vi "SendQueryMsg.vi"(0 "VISAリソース名":refnum<visa-resource-name>, 5 "入力文字列":string, 7 "タイムアウト":u32, 9 "ターミネータ":string(combo)="\n", 11 "エラー入力":errorcluster) -> (6 "受信文字列":string, 15 "エラー出力":errorcluster)   [LabVIEW 2012]
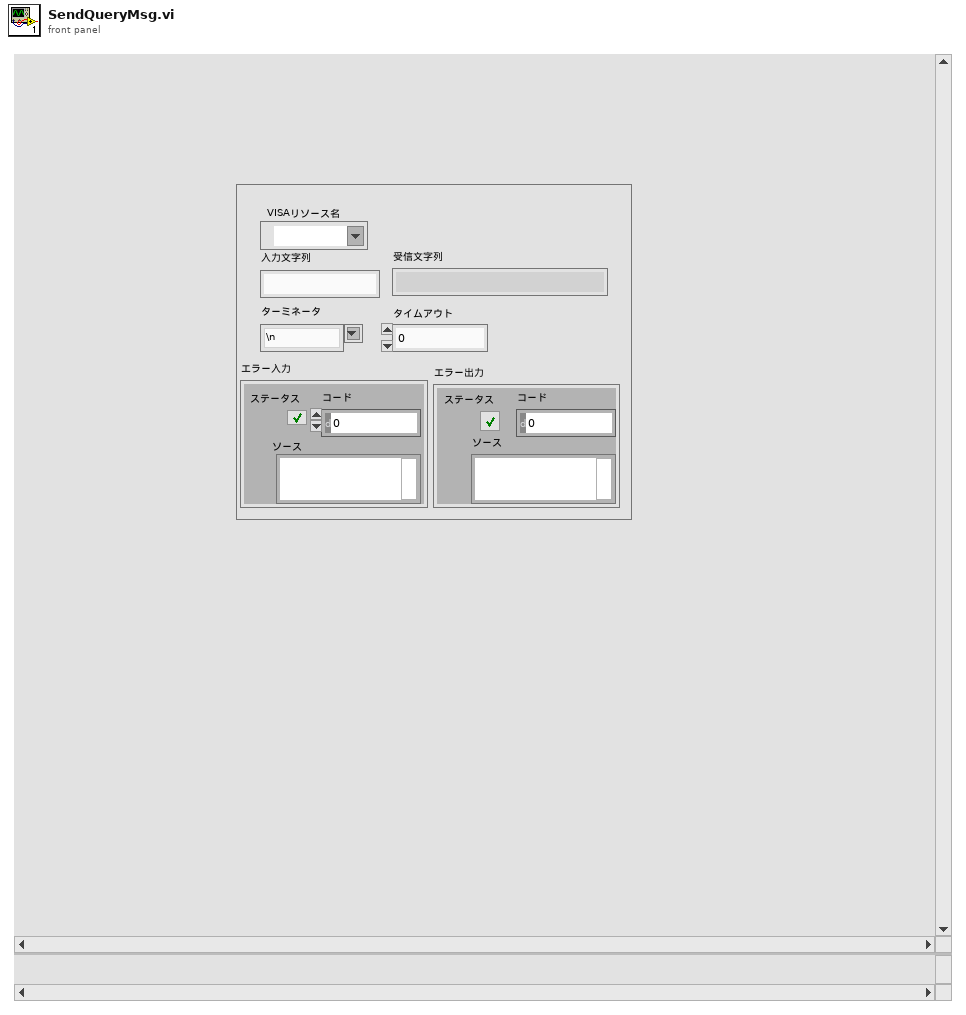
[diagram p1: front panel]
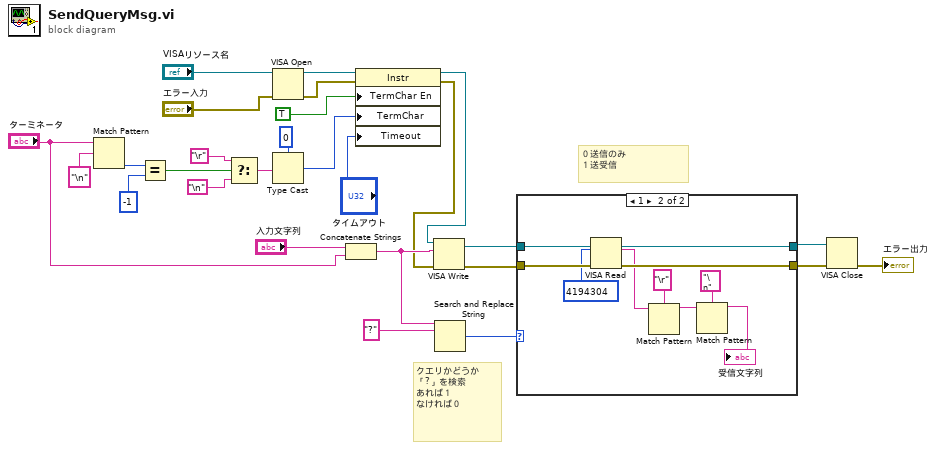
[diagram p0: block diagram]
diagram:
  # "０送信のみ\n１送受信"
  # "クエリかどうか\n「?」を検索\nあれば１\nなければ０"
  n1 = Match Pattern(string="ターミネータ", regular expression="\n" ("正規表現")) -> (offset past match=w3:i32)  [unwired: 1 in, 3 out]
  n2 = Equal?(x=w3, y=-1) -> (x = y?=w8:bool)
  n3 = Select(t="\r", s=w8, f="\n") -> (s? t:f=w9:string)
  n4 = VISA Open(error in (no error)="エラー入力", VISA resource name="VISAリソース名") -> (VISA resource name=w17:refnum<visa-resource-name>, error out=w14:errorcluster)  [unwired: 3 in]
  n5 = Type Cast(type=u8 0, x=w9) -> (*(type *) &x=w10:u8)
  n6 = Concatenate Strings("入力文字列", "ターミネータ") -> (w25:string)
  n7 = property class="Instr"(reference=w17, error in=w14, "TermChar En"=TRUE, "TermChar"=w10, "Timeout"="タイムアウト") -> (reference out=w16:refnum<visa-resource-name>, error out=w13:errorcluster)
  n8 = VISA Write(VISA resource name=w16, write buffer=w25, error in (no error)=w13) -> (VISA resource name out=w23:refnum<visa-resource-name>, error out=w21:errorcluster)  [unwired: 1 out]
  n9 = Search and Replace String(input string=w25, search string="?" ("検索文字列")) -> (number of replacements=w26:i32)  [unwired: 6 in, 3 out]
  n10 = case shown="1" w26 {
    tunnel: w21 -> [w28 w39]
    tunnel: [w29 w38] -> w24
    tunnel: w23 -> [w29 w37]
    tunnel: [w28 w35] -> w20
    frame 0, Default {
    }
    frame 1 {
      n11 = VISA Read(VISA resource name=w37, byte count=4194304, error in (no error)=w39) -> (VISA resource name out=w38:refnum<visa-resource-name>, read buffer=w31:string, error out=w35:errorcluster)  [unwired: 1 out]
      n12 = Match Pattern(string=w31, regular expression="\r") -> (before substring=w34:string)  [unwired: 1 in, 3 out]
      n13 = Match Pattern(string=w34, regular expression="\n") -> (before substring=→"受信文字列":string)  [unwired: 1 in, 3 out]
    }
  }
  n14 = VISA Close(VISA resource name=w24, error in (no error)=w20) -> (error out=→"エラー出力":errorcluster)
